vi "FloatToHex.vi"(7 "转换类型":enum16{"DCBA", "CDAB"}(ring), 11 "浮点数":sgl[](array[numeric])) -> (3 "CDAB整形输出":u16[](array[numeric]) format="%04xH")   [LabVIEW 2016, in "质控单元V1.lvlib"]
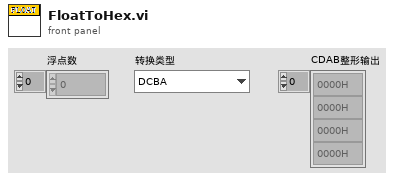
[diagram p1: front panel]
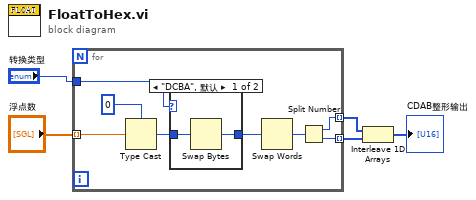
[diagram p0: block diagram]
diagram:
  n1 = for {
    tunnel: "浮点数" -> [w11] mode=indexing
    tunnel: [w10] -> w3 mode=indexing
    tunnel: [w9] -> w4 mode=indexing
    tunnel: "转换类型" -> [w8]
    n2 = Type Cast(type=0, x=w11) -> (*(type *) &x=w6:i32)
    n3 = case shown="\"DCBA\", 默认" w8 {
      tunnel: [w14 w16] -> w7
      tunnel: w6 -> [w15 w16]
      frame "DCBA", Default {
        n4 = Swap Bytes(anything=w15) -> (byte swapped=w14:i32)
      }
      frame "CDAB" {
      }
    }
    n5 = Swap Words(1:w7) -> (0:w13:i32)
    n6 = Split Number(x=w13) -> (hi(x)=w10:u16, lo(x)=w9:u16)
  }
  n7 = Interleave 1D Arrays(w3, w4) -> (→"CDAB整形输出":u16[])
